vi "GetHandles.vi"(8 "error in (no error)":errorcluster, 11 "FgenPluginsBase in":refnum<class "FgenPluginsBase.lvclass">) -> (0 "error out":errorcluster, 1 "AllHandles":string[](array[string]), 2 "FirstHandle":string, 3 "FgenPluginsBase out":refnum<class "FgenPluginsBase.lvclass">)   [LabVIEW 2018, in "FgenPlugins.lvlib" / "FgenPluginsBase.lvclass"]
uses:
  FgenPluginsBase.lvclass
  FgenPluginsBase.lvclass/FgenPluginsBase.ctl
  Accessors/Read Channels.vi
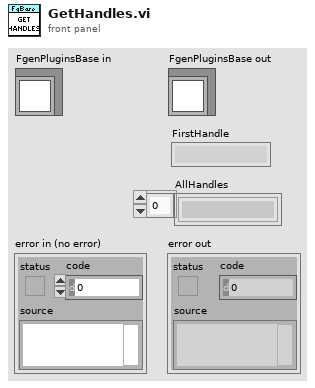
[diagram p1: front panel]
types:
  T1 = typedef "FgenPlugins.lvlib/Channel.ctl" = cluster{"Name":string, "Enabled":bool, "Operation":enum16{"Continuous", "Burst"}, "Impedance (50)":dbl, "Handle":string, "Connected":bool, "Mode (Function)":enum16{"Function", "Arbitrary", "Sequence"}}
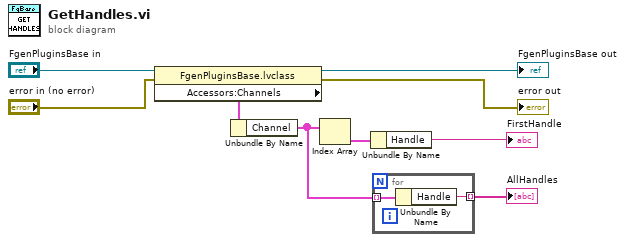
[diagram p0: block diagram]
diagram:
  n1 = property class="FgenPluginsBase.lvclass"(reference="FgenPluginsBase in", error in="error in (no error)") -> (reference out=→"FgenPluginsBase out":refnum<class "FgenPluginsBase.lvclass">, error out=→"error out":errorcluster, "Accessors:Channels"=w3:cluster{"Count":u16, "Channel":T1[]})
  n2 = Unbundle By Name(w3) -> ("Channel"=w2:T1[])
  n3 = Index Array(array=w2) -> (element=w1:T1)  [unwired: 1 in]
  n4 = Unbundle By Name(w1) -> ("Handle"=→"FirstHandle":string)
  n5 = for {
    tunnel: w2 -> [w11] mode=indexing
    tunnel: [w10] -> w4 mode=indexing
    n6 = Unbundle By Name(w11) -> ("Handle"=w10:string)
  }
  "AllHandles" <- w4
